vi "_Remote Get Leybold Error.vi"(3 "ErrorIndex (0)":u8) -> (0 "GeneratedTelegrams":string[](array[string]), 1 "Reply":string[](array[string]))   [LabVIEW 2012]
panel:
  out "ReplyParam":u32[](array[numeric])
  in  "TemplateTelegrams":string[](array[string])=["\u0002\u0016\u0000`«\u0000\u0000\u0000\u0000\u0000\u0000\u0004\u0001\u0000\u0000\u0000\u0000\u0000\u0000\u0000\u0000\u0000\u0000Ú", "\u0002\u0016\u0000`®\u0000\u0000\u0000\u0000\u0000\u0000\u0004\u0001\u0000\u0000\u0000\u0000\u0000\u0000\u0000\u0000\u0000\u0000ß", "\u0002\u0016\u0000`°\u0000\u0000\u0000\u0000\u0000\u0000\u0004\u0001\u0000\u0000\u0000\u0000\u0000\u0000\u0000\u0000\u0000\u0000Á"]
  # "Index"
  # "Error #"
  # "Description"
  # "For Error #"
  # "Freq. (Hz)"
  # "For Freq (Hz)"
  # "Time (hr)"
  # "For Time (hr)"
  # "Cause"
  # "Remedy"
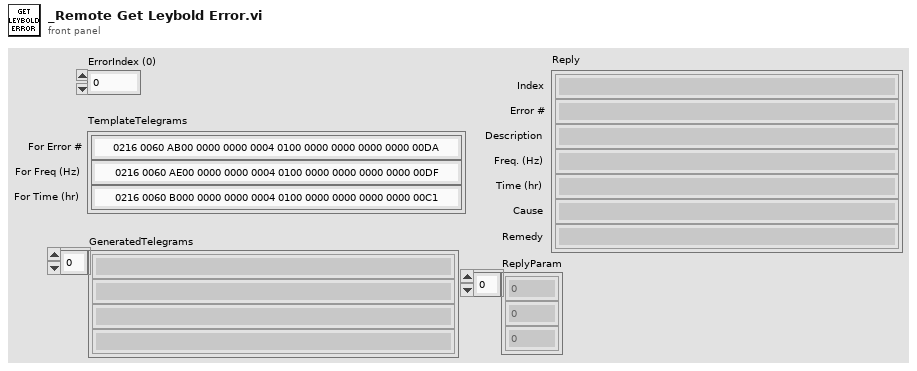
[diagram p1: front panel]
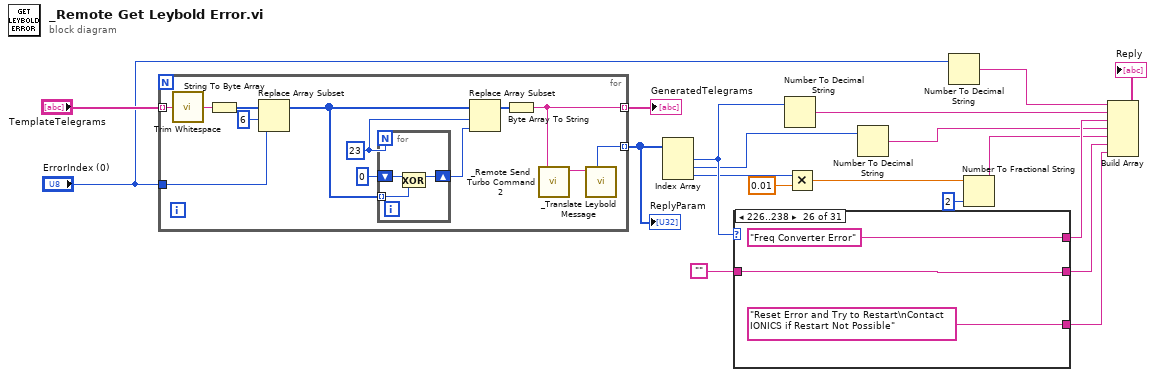
[diagram p0: block diagram]
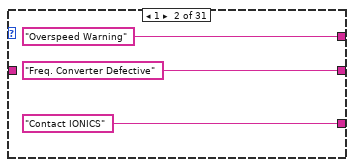
[diagram p3: hidden frame]
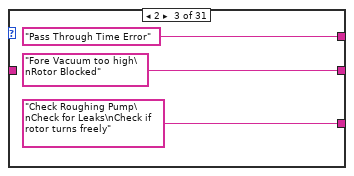
[diagram p4: hidden frame]
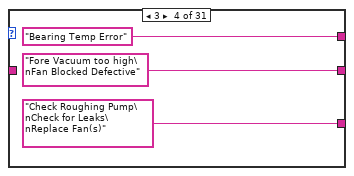
[diagram p5: hidden frame]
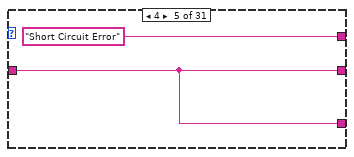
[diagram p6: hidden frame]
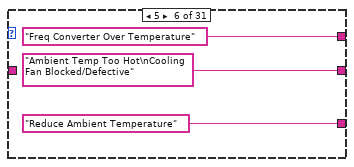
[diagram p7: hidden frame]
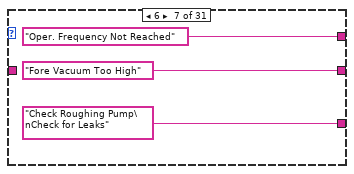
[diagram p8: hidden frame]
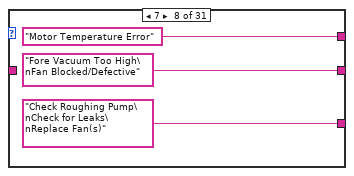
[diagram p9: hidden frame]
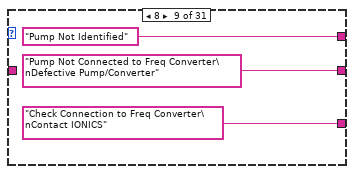
[diagram p10: hidden frame]
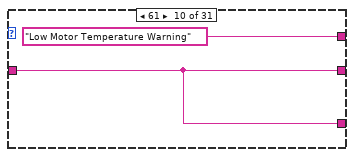
[diagram p11: hidden frame]
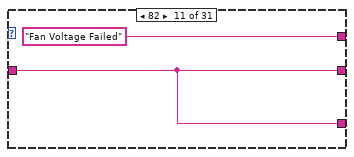
[diagram p12: hidden frame]
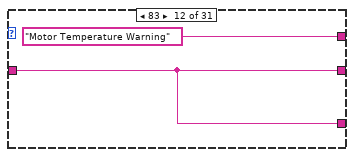
[diagram p13: hidden frame]
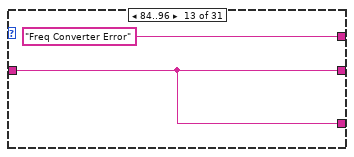
[diagram p14: hidden frame]
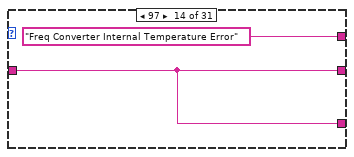
[diagram p15: hidden frame]
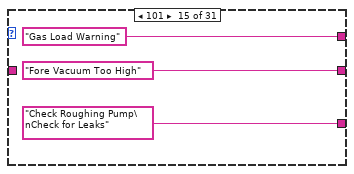
[diagram p16: hidden frame]
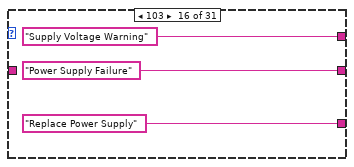
[diagram p17: hidden frame]
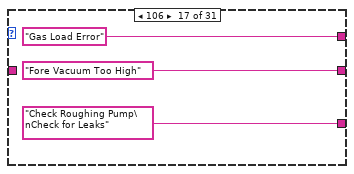
[diagram p18: hidden frame]
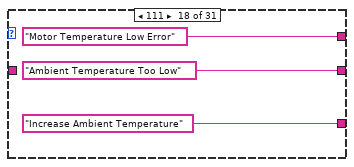
[diagram p19: hidden frame]
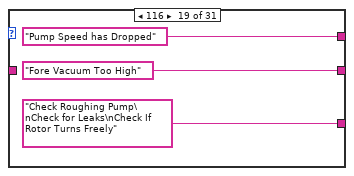
[diagram p20: hidden frame]
diagram:
  n1 = for {
    tunnel: [w26] -> w19 mode=indexing
    tunnel: "TemplateTelegrams" -> [w23] mode=indexing
    tunnel: "ErrorIndex (0)" -> [w21]
    tunnel: [w20] -> w17 mode=indexing
    w30 = 23
    n2 = call <vilib>:"Trim Whitespace.vi"("string"=w23) -> ("trimmed string"=w24:string)  [unwired: 1 in]
    n3 = String To Byte Array(string=w24) -> (unsigned byte array=w22:u8[])
    n4 = Replace Array Subset(array=w22, new element=w21, index=6) -> (w28:u8[])
    n5 = for {
      N: w30 -> [_]
      tunnel: w28 -> [w34] mode=indexing
      shift-right: [w33] -> w29
      shift-left: u8 0 -> [w35]
      n6 = Exclusive Or(1:w34, 2:w35) -> (0:w33:u8)
    }
    n7 = Replace Array Subset(array=w28, new element=w29, index=w30) -> (w27:u8[])
    n8 = Byte Array To String(unsigned byte array=w27) -> (string=w26:string)
    n9 = call "_Remote Send Turbo Command 2.vi"("Telegram"=w26) -> ("Raw Reply"=w25:string)  [unwired: 5 in, 1 out]
    n10 = call "_Translate Leybold Message.vi"("LeyboldMessage"=w25) -> ("Parameter"=w20:u32)  [unwired: 3 in, 7 out]
  }
  "GeneratedTelegrams" <- w19
  "ReplyParam" <- w17
  n11 = Index Array(array=w17) -> (element #1=w13:u32, element #2=w10:u32, element #3=w8:u32)  [unwired: 3 in]
  n12 = case shown="226..238" w13 {
    tunnel: "" -> [w36 _ _ _ w46 _ _ _ _ w60 w62 w64 w66 w68 _ _ _ _ _ _ _ _ w94 w96 _ w102 w105 _ w110 w113 w116]
    tunnel: [w36 "Overspeed Warning" "Pass Through Time Error" "Bearing Temp Error" "Short Circuit Error" "Freq Converter Over Temperature" "Oper. Frequency Not Reached" "Motor Temperature Error" "Pump Not Identified" "Low Motor Temperature Warning" "Fan Voltage Failed" "Motor Temperature Warning" "Freq Converter Error" "Freq Converter Internal Temperature Error" "Gas Load Warning" "Supply Voltage Warning" "Gas Load Error" "Motor Temperature Low Error" "Pump Speed has Dropped" "Motor Current Too Low At Startup" "Defective Bearing Temperature Sensor" "Defective Motor Temperature Sensor" "Overspeed Error" "Bearing Break-in Function Active" "Temperature Derating Active" "Freq Converter Error" "EEPROM Error" "Hardware Plausibility Error" "Inside Volume Temperature Warning" "Inside Volume Temperature Error" "Intermediate Circuit Voltage Warning"] -> w11
    tunnel: [w36 "Freq. Converter Defective" "Fore Vacuum too high\nRotor Blocked" "Fore Vacuum too high\nFan Blocked Defective" w46 "Ambient Temp Too Hot\nCooling Fan Blocked/Defective" "Fore Vacuum Too High" "Fore Vacuum Too High\nFan Blocked/Defective" "Pump Not Connected to Freq Converter\nDefective Pump/Converter" w60 w62 w64 w66 w68 "Fore Vacuum Too High" "Power Supply Failure" "Fore Vacuum Too High" "Ambient Temperature Too Low" "Fore Vacuum Too High" "Cable/Connector Faulty" "Defective Component, Short Circuit/Broken" "Defective Component, Short Circuit/Broken" w94 w96 "Temperature Sensor Threshold Exceeded,\nPump's Max Current Was Reduced for Safety" w102 w105 "Pump and Frequency Converter are\nNot Compatible" w110 w113 w116] -> w3
    tunnel: [w36 "Contact IONICS" "Check Roughing Pump\nCheck for Leaks\nCheck if rotor turns freely" "Check Roughing Pump\nCheck for Leaks\nReplace Fan(s)" w46 "Reduce Ambient Temperature" "Check Roughing Pump\nCheck for Leaks" "Check Roughing Pump\nCheck for Leaks\nReplace Fan(s)" "Check Connection to Freq Converter\nContact IONICS" w60 w62 w64 w66 w68 "Check Roughing Pump\nCheck for Leaks" "Replace Power Supply" "Check Roughing Pump\nCheck for Leaks" "Increase Ambient Temperature" "Check Roughing Pump\nCheck for Leaks\nCheck If Rotor Turns Freely" "Check Power Connections\nContact IONICS" "Contact IONICS" "Contact IONICS" w94 "Disable Break-in Function" "Determine the Temperature Fault to \nTroubleshoot the Solution" "Reset Error and Try to Restart\nContact IONICS if Restart Not Possible" w105 "Ensure Compatibility Between Pump and\nFrequency Converter" "Improve Cooling" "Improve Cooling" w116] -> w2
    frame 0, Default {
    }
    frame 1 {
    }
    frame 2 {
    }
    frame 3 {
    }
    frame 4 {
    }
    frame 5 {
    }
    frame 6 {
    }
    frame 7 {
    }
    frame 8 {
    }
    frame 61 {
    }
    frame 82 {
    }
    frame 83 {
    }
    frame 84..96 {
    }
    frame 97 {
    }
    frame 101 {
    }
    frame 103 {
    }
    frame 106 {
    }
    frame 111 {
    }
    frame 116 {
    }
    frame 117 {
    }
    frame 126 {
    }
    frame 128 {
    }
    frame 143 {
    }
    frame 144 {
    }
    frame 225 {
    }
    frame 226..238 {
    }
    frame 240 {
    }
    frame 252 {
    }
    frame 610 {
    }
    frame 611 {
    }
    frame 612 {
    }
  }
  n13 = Number To Decimal String(number=w13) -> (decimal integer string=w12:string)  [unwired: 1 in]
  n14 = Multiply(x=w8, y=0.01) -> (x*y=w6:dbl)
  n15 = Number To Decimal String(number=w10) -> (decimal integer string=w9:string)  [unwired: 1 in]
  n16 = Number To Decimal String(number="ErrorIndex (0)") -> (decimal integer string=w14:string)  [unwired: 1 in]
  n17 = Number To Fractional String(number=w6, precision (6)=i16 2) -> (F-format string=w5:string)  [unwired: 2 in]
  n18 = Build Array(w14, w12, w11, w9, w5, w3, w2) -> (→"Reply":string[])
